vi "Registered Groups.vi"(8 "error in (no error)":errorcluster, 11 "RemoteDataService in":refnum<class "RemoteDataService.lvclass">) -> (0 "error out":errorcluster, 2 "Registered Groups":string[](array[string]), 3 "RemoteDataService out":refnum<class "RemoteDataService.lvclass">)   [LabVIEW 2020, in "Vecto.lvlib" / "RemoteDataService.lvclass"]
uses:
  RemoteDataService.lvclass
  lv-promises/Promises/Promise/Promise.lvclass
  GroupsValue/GroupsValue.lvclass
  Registered Groups Data.ctl
  lv-promises/Promises/Future/Future.lvclass
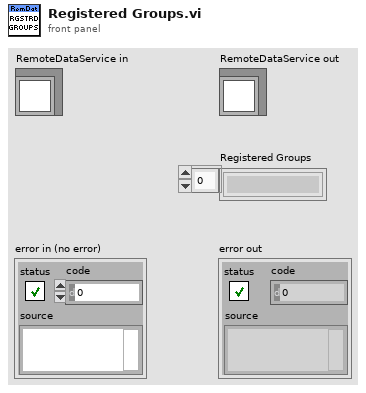
[diagram p1: front panel]
types:
  T1 = typedef "Vecto.lvlib/RemoteDataService.lvclass/Registered Groups Data.ctl" = cluster{"Promise":refnum<class "Promise.lvclass">}
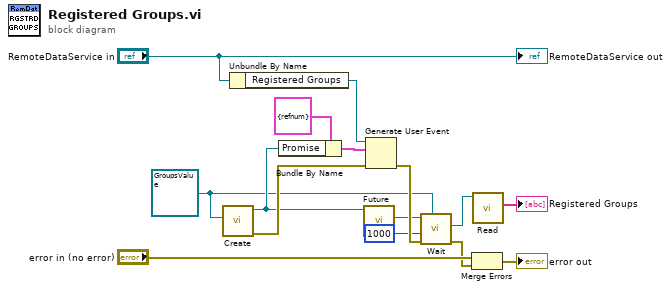
[diagram p0: block diagram]
diagram:
  w5 = refnum<class "GroupsValue.lvclass"> refnum ("Vecto.lvlib:GroupsValue.lvclass")
  n1 = call "Create.vi"("Result Type"=w5) -> ("error out"=w14:errorcluster, "Promise"=w8:refnum<class "Promise.lvclass">)  [unwired: 9 in]
  n2 = Unbundle By Name("RemoteDataService in") -> ("Registered Groups"=w11:refnum<user-event>)
  n3 = Bundle By Name(cluster=T1 {"Promise"=refnum} ("event data"), "Promise"=w8) -> (w9:T1)
  n4 = call "Future.vi"("Promise in"=w8) -> ("Future"=w7:refnum<class "Future.lvclass">)  [unwired: 9 in, 1 out]
  n5 = Generate User Event(user event=w11, event data cluster=w9, error in=w14) -> (error out=w15:errorcluster)  [unwired: 1 in, 1 out]
  n6 = call "Wait.vi"("Result Type"=w5, "error in (no error)"=w15, "Timeout mS (-1)"=1000, "Future in"=w7) -> ("error out"=w1:errorcluster, "Result"=w4:refnum<class "GroupsValue.lvclass">)  [unwired: 6 in]
  n7 = Merge Errors("error in (no error)", w1) -> (→"error out":errorcluster)
  n8 = call "Read.vi"("GroupsValue in"=w4) -> ("Groups"=→"Registered Groups":string[])  [unwired: 10 in]
  "RemoteDataService out" <- "RemoteDataService in"
